vi "insertion-sort.vi"(8 "error in":errorcluster, 11 "input":dbl[](array[numeric])) -> (0 "error out":errorcluster, 3 "output":dbl[](array[numeric]))   [LabVIEW 2016]
doc: "This is an efficient algorithm to sort arrays of a small number of elements. An <b>input</b> array with a sequence of <b>n</b> numbers in no particular order is sorted in ascending order and returned in <b>output</b>.\n\nThis VI runs the <b>insertion sort</b> algorithm introduced in topic 2.1, page 16. The pseudocode is located in page 18.\n\nCormen, T. H., Leiserson, C. E., Rivest, R. L., & Stein, C. (2009). Introduction to Algorithms (3rd ed.). Cambridge, MA: The MIT Press."
panel:
  # "INSERTION-SORT\nThis VI runs the insertion sort algorithm introduced in topic 2.1, page 16. The pseudocode is located in page 18.\nCormen, T. H., Leiserson, C. E., Rivest, R. L., & Stein, C. (2009). Introduction to Algorithms (3rd ed.). Cambridge, MA: The MIT Press.\n\nNote: in LabVIEW arrays are zero-based whereas in the book are one-based."
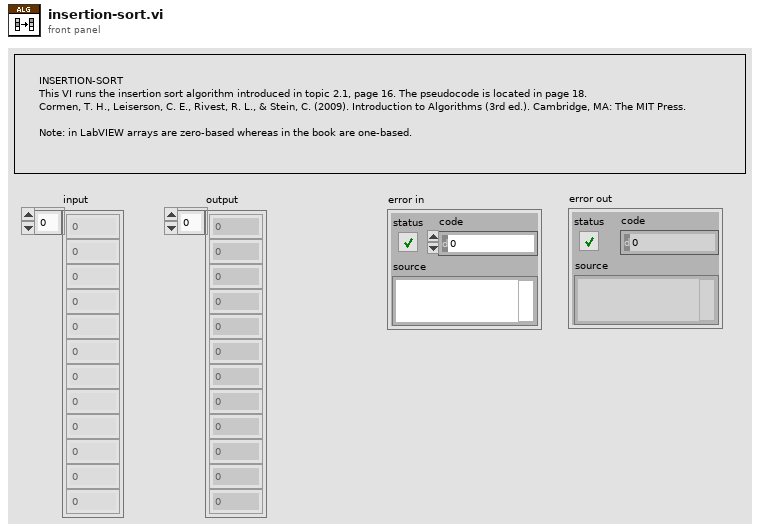
[diagram p1: front panel]
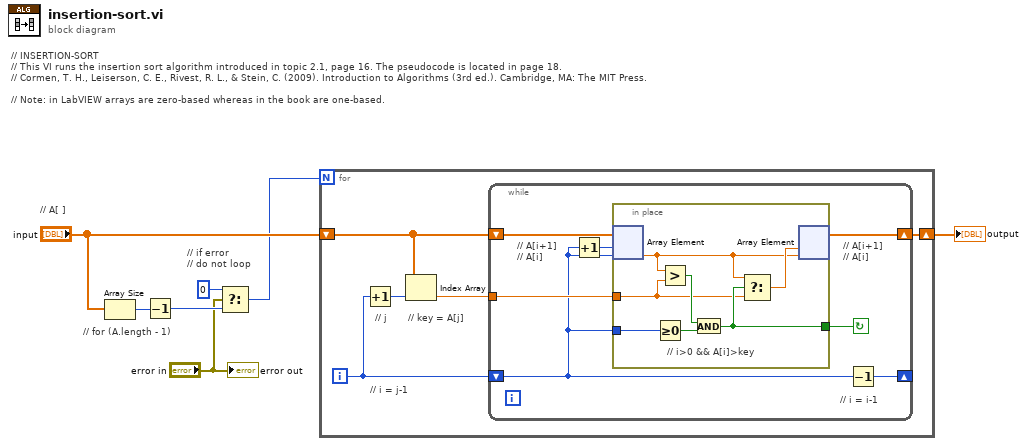
[diagram p0: block diagram]
diagram:
  # "// if error \n// do not loop"
  # "// A[ ]"
  # "// INSERTION-SORT\n// This VI runs the insertion sort algorithm introduced in topic 2.1, page 16. The pseudocode is located in page 18.\n// Cormen, T. H., Leiserson, C. E., Rivest, R. L., & Stein, C. (2009). Introduction to Algorithms (3rd ed.). Cambridge, MA: The MIT Press.\n\n// Note: in LabVIEW arrays are zero-based whereas in the book are one-based."
  # "// for (A.length - 1)"
  n1 = Array Size(array="input") -> (size(s)=w6:i32)
  n2 = Decrement(x=w6) -> (x-1=w4:i32)
  n3 = Select(t=0, s="error in", f=w4) -> (s? t:f=w3:i32)
  n4 = for {
    N: w3 -> [_]
    shift-right: [w8] -> w5
    shift-left: "input" -> [w10]
    i -> [w9]
    # "// j"
    # "// i = j-1"
    # "// key = A[j]"
    n5 = Increment(x=w9) -> (x+1=w12:i32)
    n6 = Index Array(array=w10, index=w12) -> (element=w11:dbl)
    n7 = while {
      shift-right: [w19] -> _
      shift-left: w9 -> [w15]
      tunnel: w11 -> [w17]
      shift-right: [w13] -> w8
      shift-left: w10 -> [w18]
      stop <- w14 continue-if-true
      # "// A[i+1]\n// A[i]"
      # "// i = i-1"
      # "// A[i+1]\n// A[i]"
      n8 = Increment(x=w15) -> (x+1=w16:i32)
      n9 = in-place {
        in-place-border: w17 -> [w20]
        in-place-border: w15 -> [w24]
        in-place-border: [w21] -> w14
        # "// i>0 && A[i]>key"
        n10 = in-place-array #1(w18, w16, w15) -> (w22:dbl)  [unwired: 1 out]
        n11 = Greater Or Equal To 0?(x=w24) -> (x >= 0?=w25:bool)
        n12 = Greater?(x=w22, y=w20) -> (0:w26:bool)
        n13 = And(x=w26, y=w25) -> (x .and. y?=w21:bool)
        n14 = Select(t=w22, s=w21, f=w20) -> (s? t:f=w23:dbl)
        n15 = in-place-array #1(w23, w22) -> (w13:dbl[])  [unwired: 2 out]
      }
      n16 = Decrement(x=w15) -> (x-1=w19:i32)
    }
  }
  "output" <- w5
  "error out" <- "error in"
